vi "Initialize_measurement.vi"(8 "Measurement":string, 9 "Spectrum Only?":bool, 11 "file path":path) -> (0 "error out":errorcluster, 1 "Group Name":string, 3 "tdms file out":refnum<k34>)   [LabVIEW 2019]
uses:
  SiPM_Tests_Global_Var.vi
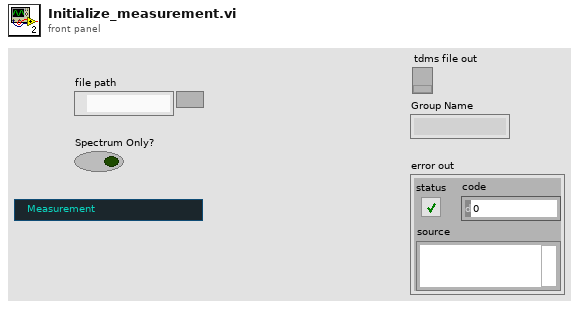
[diagram p1: front panel]
types:
  T1 = enum16{"big-endian, network order", "native, host order", "little-endian"}
  T2 = enum16{"open", "open or create", "create or replace", "create", "open (read-only)"}
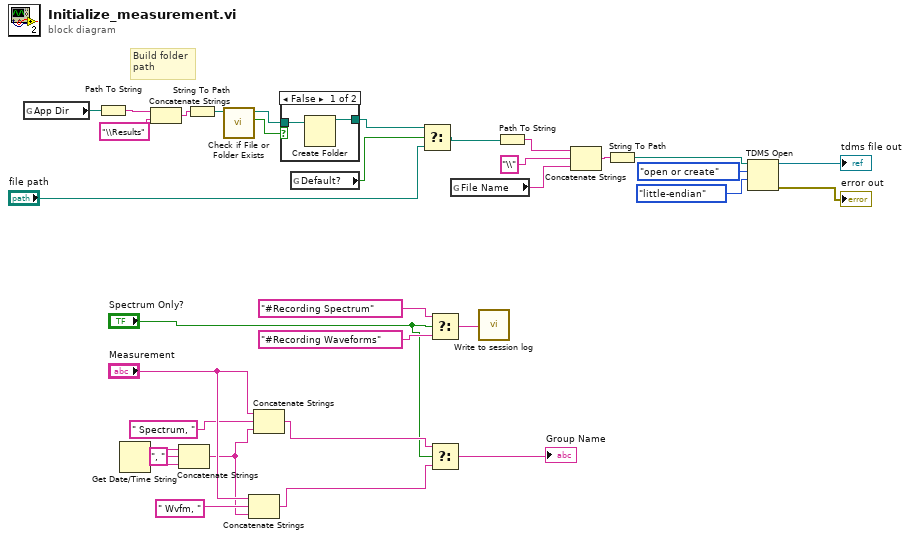
[diagram p0: block diagram]
diagram:
  # "Build folder\npath"
  n1 = global read "SiPM_Tests_Global_Var.vi" "App Dir"() -> (w15:path)
  n2 = Path To String(path=w15) -> (string=w16:string)
  n3 = Get Date/Time String() -> (date string=w30:string, time string=w28:string)  [unwired: 3 in]
  n4 = Concatenate Strings(w16, "\\Results" ("string")) -> (w14:string)
  n5 = Concatenate Strings(w30, ", " ("string"), w28) -> (w29:string)
  n6 = String To Path(string=w14) -> (path=w13:path)
  n7 = call <vilib>:"Check if File or Folder Exists.vi"("path"=w13) -> ("file or folder exists?"=w12:bool, "dup path"=w11:path)  [unwired: 8 in, 1 out]
  n8 = Concatenate Strings("Measurement", " Wvfm, " ("group name in (Untitled)"), w29) -> (w23:string)
  n9 = Concatenate Strings("Measurement", " Spectrum, " ("group name in (Untitled)"), w29) -> (w24:string)
  n10 = case shown="False" w12 {
    tunnel: [w36 w37] -> w17
    tunnel: w11 -> [w35 w37]
    frame False {
      n11 = Create Folder(path (use dialog)=w35) -> (created path=w36:path)  [unwired: 2 in, 2 out]
    }
    frame True {
    }
  }
  n12 = global read "SiPM_Tests_Global_Var.vi" "Default?"() -> (w18:bool)
  n13 = Select(t=w17, s=w18, f="file path") -> (s? t:f=w6:path)
  n14 = Select(t="#Recording Spectrum" ("Session string"), s="Spectrum Only?", f="#Recording Waveforms" ("Session string")) -> (s? t:f=w25:string)
  n15 = Select(t=w24, s="Spectrum Only?", f=w23) -> (s? t:f=→"Group Name":string)
  n16 = global read "SiPM_Tests_Global_Var.vi" "File Name"() -> (w5:string)
  n17 = call "Write to session log.vi"("Session string"=w25) -> ()  [unwired: 1 in]
  n18 = Path To String(path=w6) -> (string=w8:string)
  n19 = Concatenate Strings(w8, "\\" ("string"), w5) -> (w7:string)
  n20 = String To Path(string=w7) -> (path=w4:path)
  n21 = TDMS Open(9:T1."little-endian" ("byte order (2:little-endian)"), 10:T2."open or create" ("operation (0:open)"), 11:w4) -> (0:→"error out":errorcluster, 3:→"tdms file out":refnum<k34>)  [unwired: 4 in]
